vi "Test Not A Path.vi"(8 "error in (no error)":errorcluster) -> (0 "error out":errorcluster, 3 "Pass?":bool)   [LabVIEW 2020]
uses:
  G-Unicode/Types/UTF-8 Path/UTF-8 Path.lvclass/UTF-8 Path.ctl
  6b62e4ae-9d30-46f6-810e-6b9b7c64f0de.vi
  da08d181-0d06-47a1-bcd7-e3ded446ef48.vi
  d5a96e37-132f-4486-9ca3-8cf8b537466d.vi
  0b43944a-ca24-45bd-9c53-ff52d1a498c8.vi
  2cd82250-98a0-4f69-81c0-10e35e6ba477.vi
  7afd6289-f762-4341-965c-ebc66d055daa.vi
  G-Unicode/Private/Conversion/Text to UTF-8.vi
  G-Unicode/Private/Conversion/Polymorphic VIs/Text to UTF-8 (LabVIEW String).vi
  G-Unicode/Private/Conversion/Path as Path.vi
  G-Unicode/Private/Conversion/Polymorphic VIs/Path as Path (UTF-8 Path).vi
  G-Unicode/Private/Conversion/Polymorphic VIs/Path as Path (LabVIEW Path).vi
  G-Unicode/Types/UTF-8 Path/Read Encoded UTF-8 Path.vi
  G-Unicode/Unicode/Detect String Encoding.vi
  G-Unicode/Private/Conversion/Encoded UTF-16LE String to Encoded UTF-8 String.vi
  G-Unicode/Types/UTF-8 Path/UTF-8 Path.lvclass
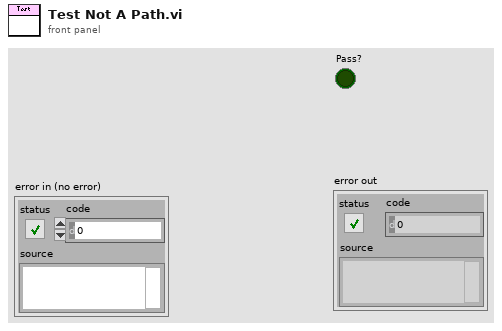
[diagram p1: front panel]
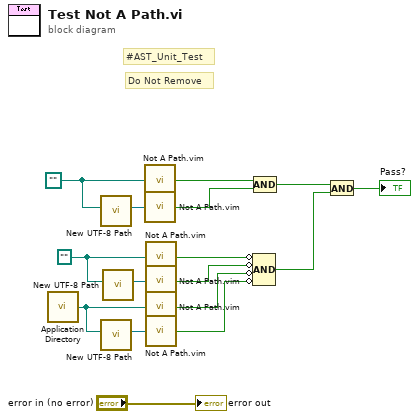
[diagram p0: block diagram]
diagram:
  w3 = path ""
  w2 = path ""
  # "Do Not Remove"
  # "#AST_Unit_Test"
  n1 = call <vilib>:"Application Directory.vi"() -> ("Application Directory"=w5:path)
  n2 = call "New UTF-8 Path.vi"("LabVIEW Path"=w2) -> ("UTF-8 Path"=w1:refnum<class "UTF-8 Path.lvclass">)  [unwired: 9 in, 1 out]
  n3 = call "New UTF-8 Path.vi"("LabVIEW Path"=w5) -> ("UTF-8 Path"=w6:refnum<class "UTF-8 Path.lvclass">)  [unwired: 9 in, 1 out]
  n4 = call "New UTF-8 Path.vi"("LabVIEW Path"=w3) -> ("UTF-8 Path"=w4:refnum<class "UTF-8 Path.lvclass">)  [unwired: 9 in, 1 out]
  n5 = call "Not A Path.vim"("Path"=w2) -> ("Path?"=w16:bool)
  n6 = call "Not A Path.vim"("Path"=w1) -> ("Path?"=w14:bool)
  n7 = call "Not A Path.vim"("Path"=w3) -> ("Path?"=w8:bool)
  n8 = call "Not A Path.vim"("Path"=w4) -> ("Path?"=w7:bool)
  n9 = call "Not A Path.vim"("Path"=w5) -> ("Path?"=w10:bool)
  n10 = call "Not A Path.vim"("Path"=w6) -> ("Path?"=w9:bool)
  n11 = Compound Arithmetic op=AND(invert w8, invert w7, invert w10, invert w9) -> (w11:bool)
  n12 = Compound Arithmetic op=AND(w16, w14) -> (w13:bool)
  n13 = And(x=w13, y=w11) -> (x .and. y?=→"Pass?":bool)
  "error out" <- "error in (no error)"
